vi "Error Query.vi"(8 "error in (no error)":errorcluster, 11 "VISA resource name":refnum<visa-resource-name>) -> (0 "error out":errorcluster, 1 "Error Message":string, 3 "VISA resource name out":refnum<visa-resource-name>)   [LabVIEW 2011, in "DMM4.lvlib"]
doc: "Queries the instrument for any errors in the instrument's error queue. It will continue to read errors until all errors have been read from the instrument. Any errors will be returned in the <B>error out</B> control.\n\n<B>Note:</B>\nThis VI is called automatically by most driver VIs so it is not usually necessary to call this in an application."
uses:
  <instrlib>/DMM4/DMM4.lvlib
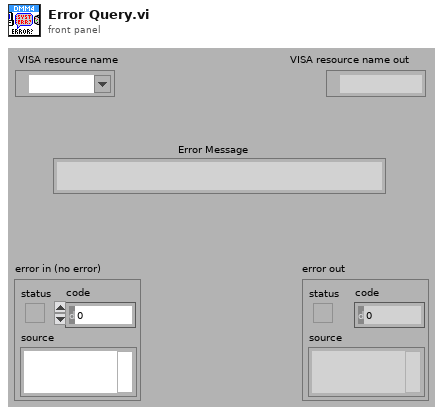
[diagram p1: front panel]
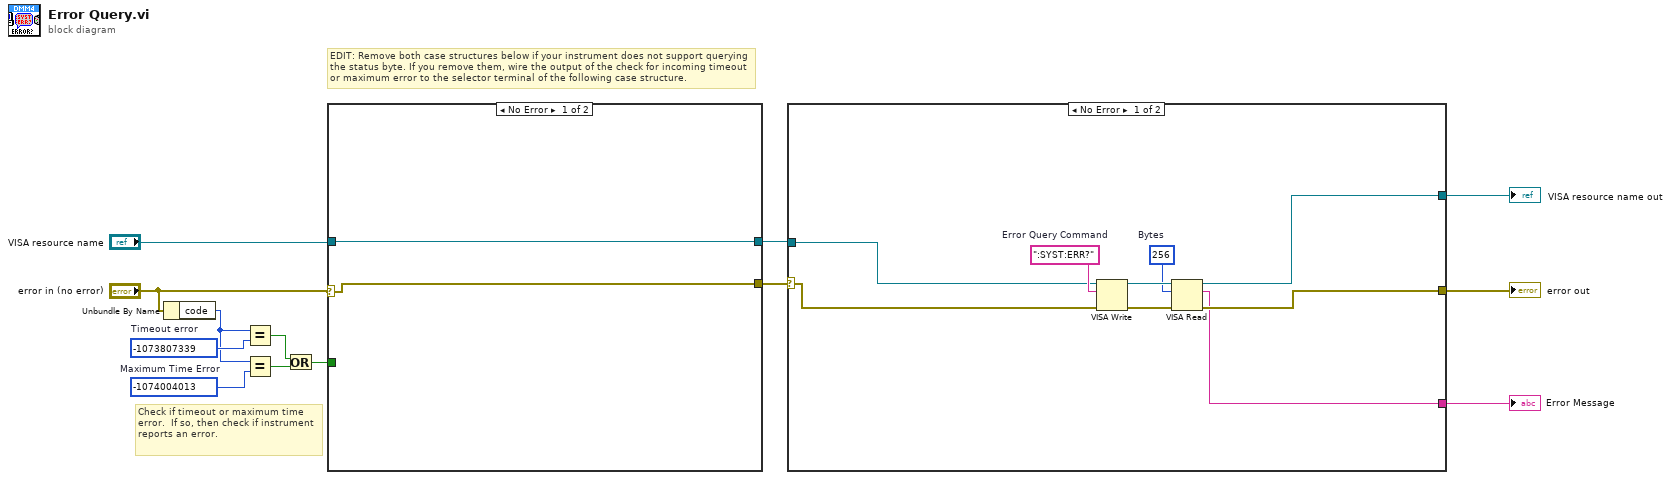
[diagram p0: block diagram]
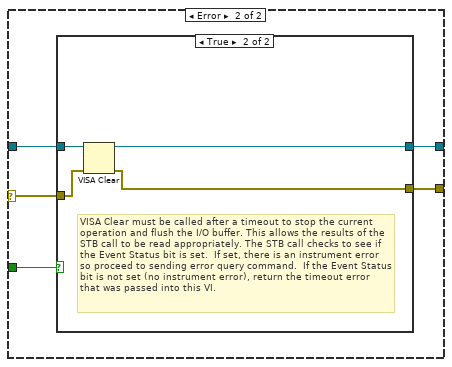
[diagram p2: hidden frame]
diagram:
  w5 = -1074004013  # Maximum Time Error
  w7 = -1073807339  # Timeout error
  # "Check if timeout or maximum time error.  If so, then check if instrument reports an error."
  # "EDIT: Remove both case structures below if your instrument does not support querying the status byte. If you remove them, wire the output of the check for incoming timeout or maximum error to the selector terminal of the following case structure."
  n1 = Unbundle By Name("error in (no error)") -> ("code"=w6:i32)
  n2 = Equal?(x=w6, y=w7) -> (x = y?=w3:bool)
  n3 = Equal?(x=w6, y=w5) -> (x = y?=w4:bool)
  n4 = Or(x=w3, y=w4) -> (x .or. y?=w2:bool)
  n5 = case shown="No Error" "error in (no error)" {
    selector: "error in (no error)" -> [w14 w16]
    tunnel: "VISA resource name" -> [w15 w20]
    tunnel: [w15 w19] -> w9
    tunnel: [w14 w18] -> w10
    tunnel: w2 -> [_ w17]
    frame No Error {
    }
    frame Error {
      n6 = case shown="True" w17 {
        tunnel: w20 -> [w22 w26]
        tunnel: [w22 w25] -> w19
        tunnel: w16 -> [w21 w24]
        tunnel: [w21 w23] -> w18
        frame False {
          # "Error code not a timeout, so best to pass on to user."
        }
        frame True {
          # "VISA Clear must be called after a timeout to stop the current operation and flush the I/O buffer. This allows the results of the  STB call to be read appropriately. The STB call checks to see if the Event Status bit is set.  If set, there is an instrument error so proceed to sending error query command.  If the Event Status bit is not set (no instrument error), return the timeout error that was passed into this VI."
          n7 = VISA Clear(VISA resource name=w26, error in (no error)=w24) -> (VISA resource name out=w25:refnum<visa-resource-name>, error out=w23:errorcluster)
        }
      }
    }
  }
  n8 = case shown="No Error" w10 {
    selector: w10 -> [w30 w36]
    tunnel: [w29 w38] -> w13
    tunnel: w9 -> [w31 w38]
    tunnel: [w28 w36] -> w12
    tunnel: [w27 ""] -> w11
    frame No Error {
      w34 = u32 256  # Bytes
      w32 = ":SYST:ERR?"  # Error Query Command
      n9 = VISA Write(VISA resource name=w31, write buffer=w32, error in (no error)=w30) -> (VISA resource name out=w35:refnum<visa-resource-name>, error out=w33:errorcluster)  [unwired: 1 out]
      n10 = VISA Read(VISA resource name=w35, byte count=w34, error in (no error)=w33) -> (VISA resource name out=w29:refnum<visa-resource-name>, read buffer=w27:string, error out=w28:errorcluster)  [unwired: 1 out]
    }
    frame Error {
    }
  }
  "VISA resource name out" <- w13
  "error out" <- w12
  "Error Message" <- w11
